vi "Read All Variables.vi"(8 "error in (no error)":errorcluster, 11 "Filter params in":refnum<class "CV-Filter.lvclass">) -> (0 "error out":errorcluster, 2 "Filter vars.":T1, 3 "Filter params out":refnum<class "CV-Filter.lvclass">)   [LabVIEW 2013, in "CameraVision.lvlib" / "CV-Filter.lvclass"]
uses:
  CV-Filter.lvclass
  Filter-variables.ctl
  Filter-settings.ctl
  Filter-characteristic.ctl
  UI/Module-states.ctl
  CV-Filter.lvclass/CV-Filter.ctl
  UI/CV-UI.lvclass
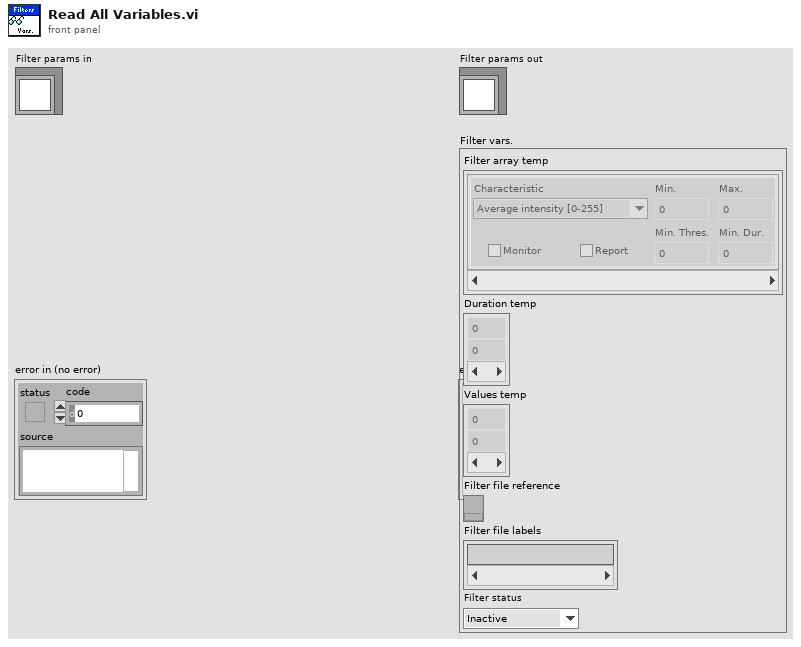
[diagram p1: front panel]
types:
  T1 = typedef "CameraVision.lvlib/CV-Filter.lvclass/Filter-variables.ctl" = cluster{"Filter array temp":T2[], "Duration temp":u16[][], "Values temp":dbl[][], "Filter file reference":refnum<k34>, "Filter file labels":string[], "Filter status":T4}
  T2 = typedef "CameraVision.lvlib/CV-Filter.lvclass/Filter-settings.ctl" = cluster{"Characteristic":T3, "Monitor":bool, "Min.":dbl, "Max.":dbl, "Min. Thres.":dbl, "Min. Dur.":u16, "Report":bool}
  T3 = typedef "CameraVision.lvlib/CV-Filter.lvclass/Filter-characteristic.ctl" = enum16{"Average intensity [0-255]", "Peak intensity [0-255]", "Melt-pool size [mm²]", "Melt-pool aspect ratio []", "Melt-pool fragments []", "Melt-pool position X [pixel]", "Melt-pool position Y [pixel]", "Average temperature [°C]", "Max. temperature [°C]", "Min. temperature [°C]", "Std. dev. temperature [°C]"}
  T4 = typedef "CameraVision.lvlib/CV-UI.lvclass/Module-states.ctl" = enum16{"Inactive", "Active", "Data-loss", "Error", "Simulation", "Synchronizing", "Initialized", "Released"}
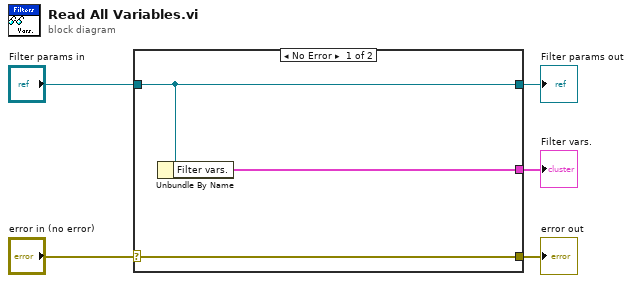
[diagram p0: block diagram]
diagram:
  n1 = case shown="No Error" "error in (no error)" {
    selector: "error in (no error)" -> [w8 w9]
    tunnel: [w8 w9] -> w4
    tunnel: [w7 w10] -> w2
    tunnel: "Filter params in" -> [w7 w10]
    tunnel: [w6 _] -> w1
    frame No Error {
      n2 = Unbundle By Name(w7) -> ("Filter vars."=w6:T1)
    }
    frame Error {
    }
  }
  "error out" <- w4
  "Filter params out" <- w2
  "Filter vars." <- w1
